vi "dsdll_capture_get_size.vi"(8 "error in":errorcluster, 10 "samples count":u32, 11 "dsdll instance in":T2={"dsdll path"=path "E:/LVprog/DirectSoundDLL/dsdll.dll", "dsdll handle"=[], "output devices"=[], "capture devices"=[]}) -> (0 "error out":errorcluster, 1 "channels count":u16, 2 "capture buffer size [B]":u32, 3 "dsdll instance out":T2, 4 "format":T1, 6 "total sample size [B]":i32)   [LabVIEW 2018, in "dsdll.lvlib"]
doc: "Call this to get byte-size of buffer required for capturing of given count of samples and currently set format of the opened capture device.\nIt also returns selected format ID and count of channels.\nAlso returns total sample byte-size (for all channels)."
uses:
  dsdll.lvlib
  dsdll_instance.ctl
  dsdll_device_record.ctl
  dsdll_sample_format.ctl
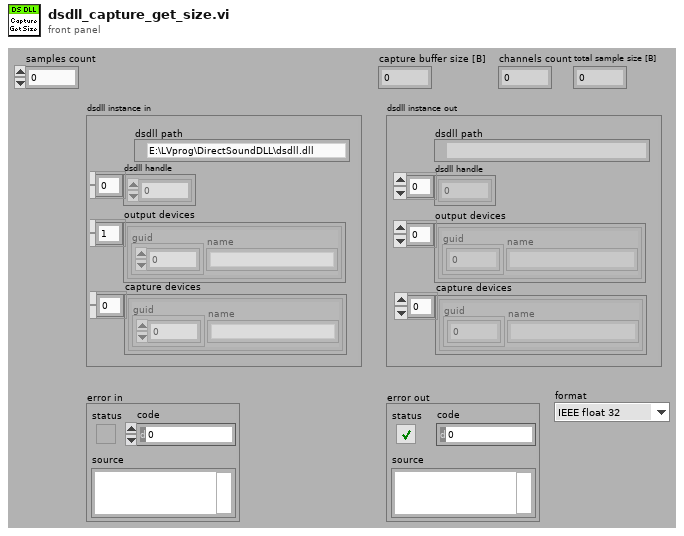
[diagram p1: front panel]
types:
  T1 = typedef "dsdll.lvlib/dsdll_sample_format.ctl" = enum16{"IEEE float 32", "PCM 16 bit"}
  T2 = typedef "dsdll.lvlib/dsdll_instance.ctl" = cluster{"dsdll path":path, "dsdll handle":u8[], "output devices":T3[], "capture devices":T3[]}
  T3 = typedef "dsdll.lvlib/dsdll_device_record.ctl" = cluster{"guid":u8[], "name":string}
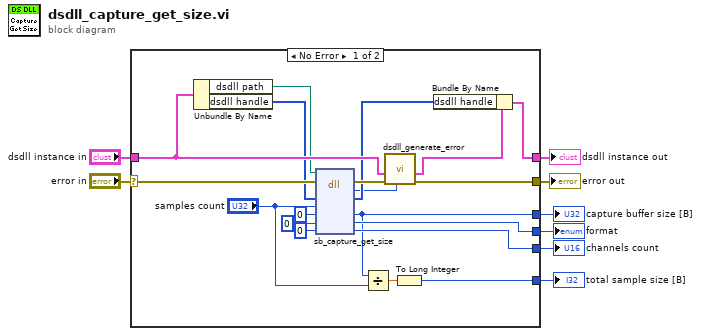
[diagram p0: block diagram]
diagram:
  n1 = case shown="No Error" "error in" {
    selector: "error in" -> [w22 w28]
    tunnel: "dsdll instance in" -> [w27 w29]
    tunnel: [w26 w28] -> w7
    tunnel: [w24 w29] -> w8
    tunnel: [w12 _] -> w4
    tunnel: [w14 _] -> w3
    tunnel: [w13 _] -> w2
    tunnel: [w9 _] -> w1
    frame No Error {
      n2 = Unbundle By Name(w27) -> ("dsdll path"=w21:path, "dsdll handle"=w20:u8[])
      n3 = dll-call lib="dsdll.dll" fn="sb_capture_get_size"(path in=w21, error in=w22, "handle"=w20, "count"="samples count", "bsize"=u32 0, "format"=u16 0, "channels"=u16 0) -> (error out=w23:errorcluster, "error"=w18:i32, "handle"=w19:u8[], "bsize"=w12:u32, "format"=w14:u16, "channels"=w13:u16)  [unwired: 2 in, 1 out]
      n4 = Divide(x=w12, y="samples count") -> (x/y=w10:dbl)
      n5 = call "dsdll_generate_error.vi"("error code"=w18, "error in"=w23, "dsdll instance in"=w27) -> ("error out"=w26:errorcluster, "dsdll instance out"=w25:T2)  [unwired: 6 in, 1 out]
      n6 = To Long Integer(number=w10) -> (32bit integer=w9:i32)
      n7 = Bundle By Name(cluster=w25, "dsdll handle"=w19) -> (w24:T2)
    }
    frame Error {
    }
  }
  "error out" <- w7
  "dsdll instance out" <- w8
  "capture buffer size [B]" <- w4
  "format" <- w3
  "channels count" <- w2
  "total sample size [B]" <- w1
